vi "Acquire.vi"(8 "error in (no error)":errorcluster, 9 "Data Queue":refnum<queue>, 10 "Data Notifier":refnum<notifier>, 11 "Hardware Resources in":T1) -> (0 "error out":errorcluster, 3 "Hardware Resources out":T1)   [LabVIEW 2019, in "Acquisition.lvlib"]
doc: "Perform the acquisition. Replace the contents of this diagram with calls to acquisition hardware."
uses:
  Acquisition.lvlib
  Hardware Configuration.ctl
  <vilib>/DAQmx/read.llb/DAQmx Read (Analog 1D Wfm NChan NSamp).vi
  <vilib>/DAQmx/miscellaneous.llb/DAQmx Fill In Error Info.vi
  <resource>/objmgr/daqmx.rc
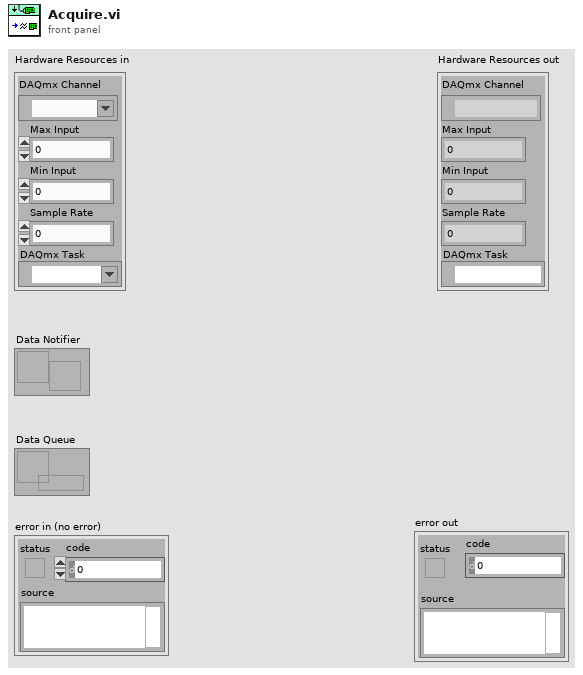
[diagram p1: front panel]
types:
  T1 = typedef "Acquisition.lvlib/Hardware Configuration.ctl" = cluster{"DAQmx Channel":tag, "Max Input":dbl, "Min Input":dbl, "Sample Rate":dbl, "DAQmx Task":refnum<k21>}
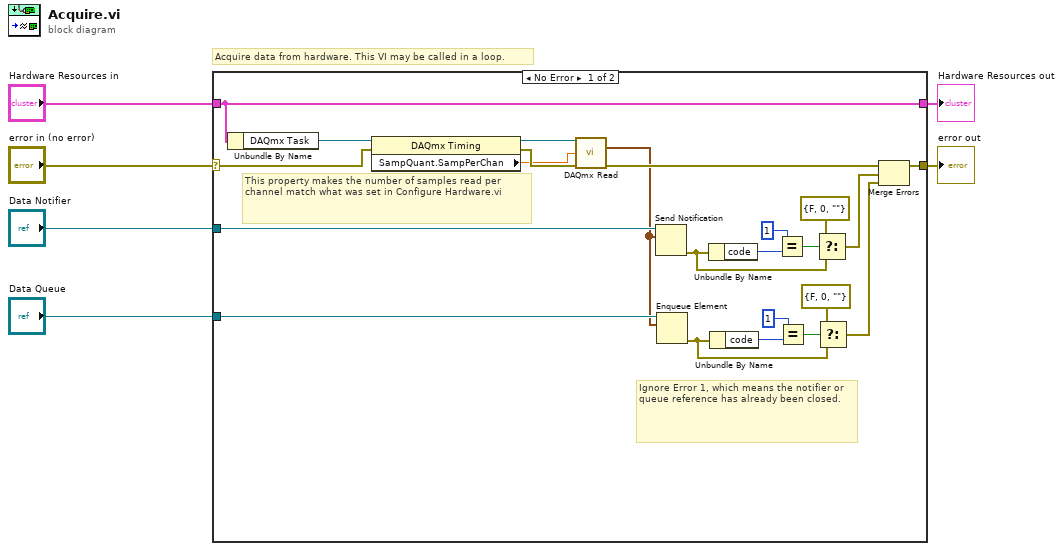
[diagram p0: block diagram]
diagram:
  # "Acquire data from hardware. This VI may be called in a loop."
  n1 = case shown="No Error" "error in (no error)" {
    selector: "error in (no error)" -> [w9 w30]
    tunnel: [w29 w30] -> w5
    tunnel: "Hardware Resources in" -> [w14 w31]
    tunnel: [w14 w31] -> w3
    tunnel: "Data Notifier" -> [w28 _]
    tunnel: "Data Queue" -> [w15 _]
    frame No Error {
      # "This property makes the number of samples read per channel match what was set in Configure Hardware.vi"
      # "Ignore Error 1, which means the notifier or queue reference has already been closed."
      n2 = Unbundle By Name(w14) -> ("DAQmx Task"=w11:refnum<k21>)
      n3 = property class="DAQmx Timing"(reference=w11, error in=w9) -> (reference out=w10:refnum<k21>, error out=w8:errorcluster, "SampQuant.SampPerChan"=w7:dbl)
      n4 = call-poly <vilib>:"DAQmx Read.vi"("task/channels in"=w10, "number of samples per channel"=w7, "error in"=w8) -> ("data"=w12:waveform(dbl)[], "error out"=w13:errorcluster)  [unwired: 10 in, 1 out]
      n5 = Send Notification(notification=w12, notifier=w28) -> (error out=w24:errorcluster)  [unwired: 1 in, 1 out]
      n6 = Enqueue Element(queue=w15, element=w12) -> (error out=w20:errorcluster)  [unwired: 2 in, 2 out]
      n7 = Unbundle By Name(w24) -> ("code"=w27:i32)
      n8 = Unbundle By Name(w20) -> ("code"=w17:i32)
      n9 = Equal?(x=1, y=w27) -> (x = y?=w25:bool)
      n10 = Equal?(x=1, y=w17) -> (x = y?=w19:bool)
      n11 = Select(t=errorcluster {"status"=FALSE, "code"=0, "source"=""} ("error constant"), s=w25, f=w24) -> (s? t:f=w23:errorcluster)
      n12 = Select(t=errorcluster {"status"=FALSE, "code"=0, "source"=""} ("error constant"), s=w19, f=w20) -> (s? t:f=w16:errorcluster)
      n13 = Merge Errors(w13, w23, w16) -> (w29:errorcluster)
    }
    frame Error {
    }
  }
  "Hardware Resources out" <- w3
  "error out" <- w5
